vi "handle_connection.vi"(6 "Log Service":refnum<data-value>, 8 "error in (no error)":errorcluster, 10 "connection":refnum<class "Connection.lvclass">, 11 "Echo Handler in":refnum<class "Echo Handler.lvclass">) -> (0 "error out":errorcluster)   [LabVIEW 2019, in "ANODE Tests.lvlib" / "Echo Handler.lvclass"]
uses:
  Echo Handler.lvclass
  ANODE/Socket API/Connection/Connection.lvclass
  ANODE/Utility API/Log Service/Log Service.lvclass
  ANODE/Utility API/Log Service/public/level.ctl
  db0a713a-f0d1-4d9a-a177-7f6fa3a9238e.vi
  ANODE/Util/Timestamp or now.vi
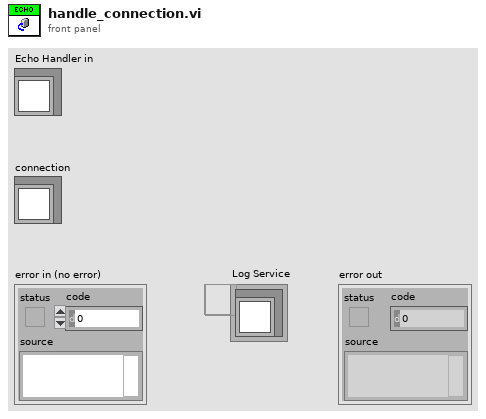
[diagram p1: front panel]
types:
  T1 = enum16{"Standard", "Buffered", "CRLF", "Immediate"}
  T2 = typedef "Utility API.lvlib/Log Service.lvclass/level.ctl" = u16
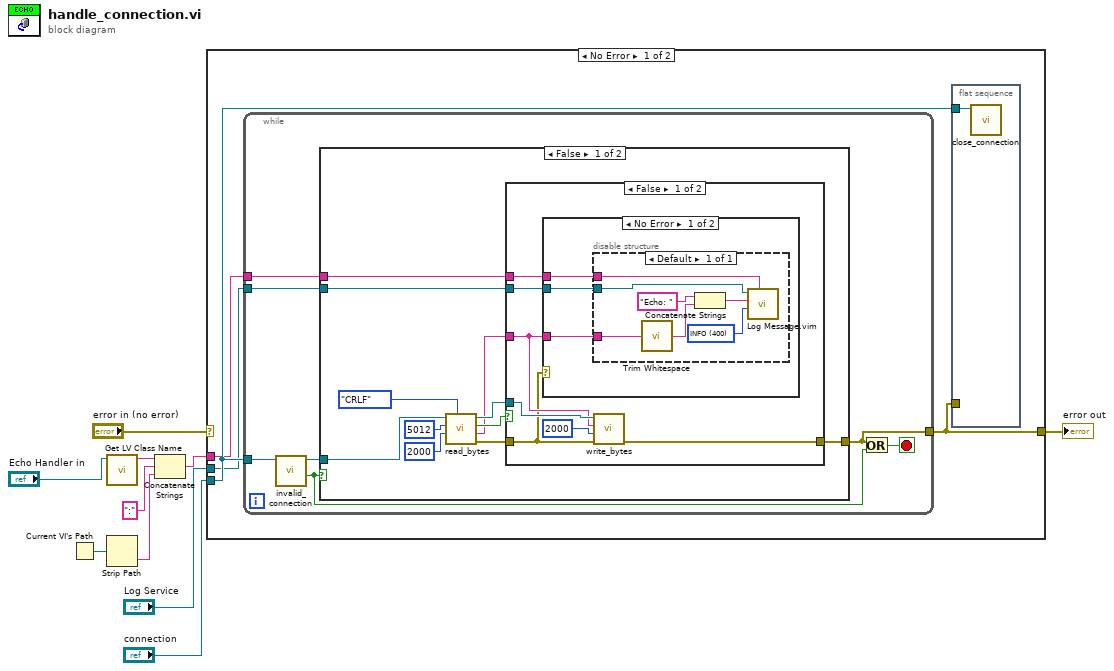
[diagram p0: block diagram]
diagram:
  n1 = Current VI's Path() -> (path=w6:path)
  n2 = call <vilib>:"Get LV Class Name.vi"("object"="Echo Handler in") -> ("class name"=w3:string)  [unwired: 9 in, 1 out]
  n3 = Strip Path(path=w6) -> (name=w4:string)  [unwired: 1 out]
  n4 = Concatenate Strings(w3, ":" ("string"), w4) -> (w2:string)
  n5 = case shown="No Error" "error in (no error)" {
    selector: "error in (no error)" -> [_ w52]
    tunnel: "connection" -> [w14 _]
    tunnel: [w13 w52] -> w8
    tunnel: "Log Service" -> [w12 _]
    tunnel: w2 -> [w11 _]
    frame No Error {
      n6 = while {
        tunnel: w14 -> [w22]
        tunnel: [w18] -> w13
        tunnel: w12 -> [w17]
        tunnel: w11 -> [w16]
        stop <- w19 stop-if-true
        n7 = call-dynamic "invalid_connection.vi"("Connection in"=w22) -> ("invalid connection?"=w20:bool, "Connection out"=w21:refnum<class "Connection.lvclass">)  [unwired: 8 in, 1 out]
        n8 = case shown="False" w20 {
          tunnel: w21 -> [w27 _]
          tunnel: [w26 _] -> w18
          tunnel: w17 -> [w24 _]
          tunnel: w16 -> [w23 _]
          frame False {
            n9 = call-dynamic "read_bytes.vi"("read mode"=T1."CRLF", "timeout (ms)"=2000, "bytes to read"=5012, "Connection in"=w27) -> ("error out"=w28:errorcluster, "data out"=w25:string, "timeout?"=w30:bool, "Connection out"=w29:refnum<class "Connection.lvclass">)  [unwired: 4 in]
            n10 = case shown="False" w30 {
              tunnel: w29 -> [w40 _]
              tunnel: w25 -> [w35 _]
              tunnel: [w38 w51] -> w26
              tunnel: w28 -> [w34 w51]
              tunnel: w24 -> [w37 _]
              tunnel: w23 -> [w36 _]
              frame False {
                n11 = case shown="No Error" w34 {
                  tunnel: w37 -> [w43 _]
                  tunnel: w36 -> [w42 _]
                  tunnel: w35 -> [w41 _]
                  frame No Error {
                    n12 = disable-structure shown="Default" {
                      disable-tunnel: w43 -> [w50]
                      disable-tunnel: w42 -> [w49]
                      disable-tunnel: w41 -> [w47]
                      frame Enabled {
                        w45 = T2 400 items=["OFF"=0, "FATAL"=100, "ERROR"=200, "WARN"=300, "INFO"=400, "DEBUG"=500, "TRACE"=600, "ALL"=65535] ("level")
                        n13 = call <vilib>:"Trim Whitespace.vi"("string"=w47) -> ("trimmed string"=w44:string)  [unwired: 1 in]
                        n14 = Concatenate Strings("Echo: ", w44) -> (w46:string)
                        n15 = call "Log Message.vim"("context"=w49, "level"=w45, "message"=w46, "Log Service in"=w50) -> ()  [unwired: 6 in, 2 out]
                      }
                    }
                  }
                  frame Error {
                  }
                }
                n16 = call-dynamic "write_bytes.vi"("error in (no error)"=w34, "timeout ms (-1)"=2000, "data in"=w35, "Connection in"=w40) -> ("error out"=w38:errorcluster)  [unwired: 4 in, 3 out]
              }
              frame True {
              }
            }
          }
          frame True {
          }
        }
        n17 = Or(x=w18, y=w20) -> (x .or. y?=w19:bool)
      }
      n18 = flat-sequence {
        tunnel: w14 -> [w15]
        tunnel: w13 -> [_]
        frame #0 {
          n19 = call-dynamic "close_connection.vi"("Connection in"=w15) -> ()  [unwired: 10 in, 1 out]
        }
      }
    }
    frame Error {
    }
  }
  "error out" <- w8
